vi "For Debug.vi"() -> ()   [LabVIEW 2015]
uses:
  AOP/Interface/CRDS/Controls/Ringdown Xctl/Ringdown.xctl
  Devices/Alicat/Session Based/Data/Alicat Data.lvclass
  Reusable/Data/Array Data/Single 1-D/Single_Array.lvclass
  Devices/TE Cooler/Data/TECData.lvclass
  Devices/TE Cooler/Data/TECData.lvclass/TECData.ctl
  Reusable/CRDS/Data/Main/CRDS Data.lvclass
  Reusable/CRDS/Data/Cell/CRDS Cell Data.lvclass/CRDS Cell Data.ctl
  Reusable/PAS/Data/Main/PAS Data.lvclass
  Reusable/PAS/Data/Cell/PAS Cell Data.lvclass
  Devices/TE Cooler/Data/Data Access/Read Input 1.vi
  Devices/TE Cooler/Data/Data Access/Read Input 2.vi
  Devices/TE Cooler/Data/Data Access/Read Power.vi
  Reusable/CRDS/Data/Cell/Read extParam.vi
  Reusable/CRDS/Data/Main/Read filter.vi
  Reusable/CRDS/Data/Main/Read CellData.vi
  Reusable/Data/Read measTime.vi
  Reusable/CRDS/Data/Cell/Read Ringdowns.vi
  Reusable/PAS/Data/Main/Write Current Cell.vi
  Reusable/PAS/Data/Main/Read Cell Frequency Data.vi
  Reusable/PAS/Data/Main/Read Cell Laser Diode Signal.vi
  Reusable/PAS/Data/Main/Read Cell Microphone Signal.vi
  Reusable/PAS/Data/Main/Read O3 flag.vi
  Reusable/PAS/Data/Main/Read CellData.vi
  Reusable/PAS/Data/Cell/Read derived.vi
  Reusable/Data/Array Data/Single 1-D/Read Data.vi
  Reusable/CRDS/Data/Cell/CRDS Cell Data.lvclass
panel:
  in  "Tab Control":enum32{"CRDS", "PAS", "TEC", "Housekeeping"}(tab)
  in  "PMT":bool
  in  "Rep Rate":i32(ring)=250 items=["1000"=1000, "500"=500, "250"=250]
  out "max":cluster{"[0]":sgl, "[1]":sgl}(graph)
  out "tau":cluster{"[0]":dbl, "[1]":dbl}(graph)
  out "Cell 1":T1 {"max" format="%#.6g"; "Tau0" format="%#.6g"; "TauCorr" format="%#.6g"; "etau" format="%#.6g"; "stdDevtau" format="%#.6g"; "extCorr" format="%#.6g"; "ext" format="%#.6g"; "Tau0Corr" format="%#.6g"; "Tau" format="%#.6g"}
  out "Cell 0":T1 {"max" format="%#.6g"; "Tau0" format="%#.6g"; "TauCorr" format="%#.6g"; "etau" format="%#.6g"; "stdDevtau" format="%#.6g"; "extCorr" format="%#.6g"; "ext" format="%#.6g"; "Tau0Corr" format="%#.6g"; "Tau" format="%#.6g"}
  in  "Num Samples per Cycle":dbl
  out "Ringdown":i16[][][](xcontrol)
  out "CRDS Time":timestamp format="%<%H:%M:%S%2u>T"
  out "Phase":dbl(graph)
  out "PAS Time":timestamp format="%<%H:%M:%S%2u>T"
  out "f0":sgl(graph)
  out "IA":sgl(graph)
  out "PAS Data":T2
  in  "Chirp Bandwidth":i16
  in  "Chirp fcenter":i16
  out "Laser Diode":waveform(i16)(graph)
  out "Frequency":waveform(sgl)(graph)
  out "Microphone":waveform(i16)(graph)
  in  "f0":dbl
  in  "DC":dbl
  in  "Vrange":dbl
  in  "Voffset":dbl
  in  "VspkParam":dbl[](array[numeric])
  in  "Speaker":bool
  in  "Modulation":dbl
  out "O3 Flag":bool
  in  "PAS TEC Power":bool
  in  "Main TEC Power":bool
  out "TEC Out":cluster{"[0]":sgl, "[1]":sgl}(graph)
  out "PAS":T3
  out "Main":T3
  in  "Tpas":sgl
  in  "Tmain":sgl
  in  "FanIn":bool
  in  "Alicat Names":string[](array[string])=["Pressure", "PAS", "CRD1", "Purge", "Ozone"]
  out "RH":cluster{"Numeric":sgl, "Numeric":sgl}(graph)
  out "T":cluster{"Numeric":sgl, "Numeric":sgl}(graph)
  out "P":T4(graph)
  in  "Solenoid  In":u8
  out "PPT 3":cluster{"P":dbl, "T":dbl}
  out "PPT 2":cluster{"P":dbl, "T":dbl}
  out "PPT 1":cluster{"P":dbl, "T":dbl}
  out "PAS":cluster{"RH":dbl, "T":dbl, "Td":dbl}
  out "CRD":cluster{"RH":dbl, "T":dbl, "Td":dbl}
  in  "Qsp":dbl[](array[numeric])
  in  "Pump":bool
  in  "Filter":bool
  out "Filter Out":bool
  out "Alicat Data":sgl[][](array[numeric])
  # "Number of samples in a single cylce refers to the number of samples that will be acquired during a ringdown.  The data acquisition is at 1 MHz, so if the value is 500, then the system is acquiring 500 us of samples per ringdown."
  # "The Rep Rate actually refers to the number of clock ticks between ringdowns.  The clock rate is 1 MHz, so if the value is 1000, there is 1000 us between each ringdown and laser is modulating at 1 kHz.  If the value is 2000,  then there are 2000 us between ringdowns and the laser is modulating at 500 Hz."
  # "Laser"
  # "Speaker"
  # "Alicat's are currently entered as follows:\nID                 Address   Controller?   Type                 Range\nPressure          A                Y                  Pressure           0-1000 \nPAS                  D                Y                  Mass                 0-5\nCRD1                B                Y                  Mass                 0-1\nPurge               E                Y                   Mass                 0-100\nOzone              F                 Y                  Volumetric       0-5"
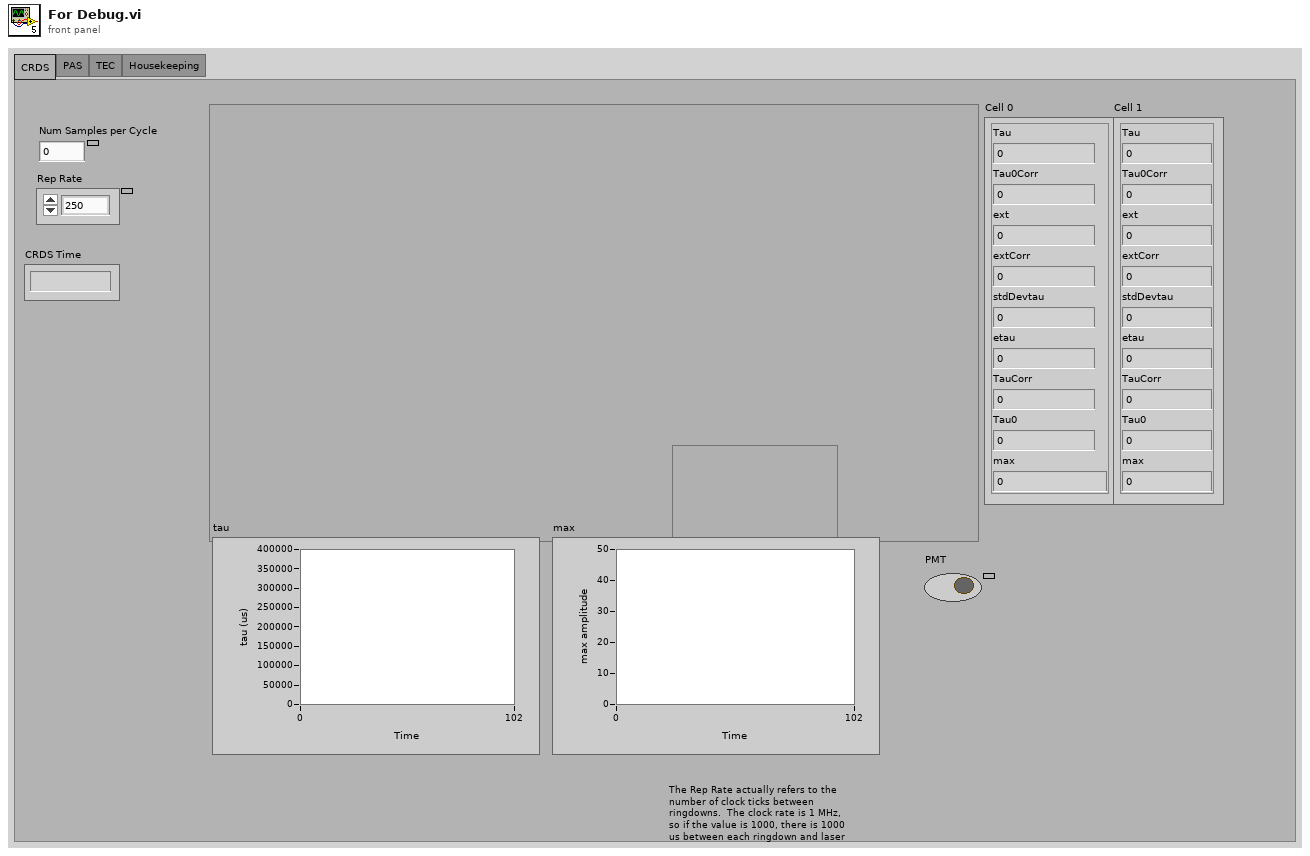
[diagram p1: front panel]
types:
  T1 = cluster{"Tau":dbl, "Tau0Corr":dbl, "ext":dbl, "extCorr":dbl, "stdDevtau":dbl, "etau":dbl, "TauCorr":dbl, "Tau0":dbl, "max":dbl}
  T2 = cluster{"f0 (Hz":dbl, "IA":dbl, "Noise Limit":dbl, "Q":dbl, "phase":dbl}
  T3 = cluster{"Input 1":dbl, "Input 2":dbl, "Power":dbl}
  T4 = cluster{"Numeric":sgl, "Numeric":sgl, "Numeric":sgl}
  T5 = cluster{"f0":sgl, "IA":sgl, "Q":sgl, "max":dbl[], "deltaPhi":dbl, "tau":dbl, "noiseLim":dbl, "ext":dbl}
  T6 = cluster{"f0":sgl, "IA":sgl, "noiseLim":dbl, "Q":sgl, "deltaPhi":dbl}
  T7 = typedef "extparam.ctl" = cluster{"Tau":sgl, "Tau0cor":sgl, "ext":sgl, "extCorr":sgl, "stdevTau":sgl, "eTau":sgl, "taucorr":sgl, "Tau0":sgl, "max":sgl}
  T8 = cluster{"Data Access:Input 1":sgl, "Data Access:Input 2":sgl, "Data Access:Power":sgl}
  T9 = cluster{"Data[0]":sgl, "Data[1]":sgl, "Data[2]":sgl}
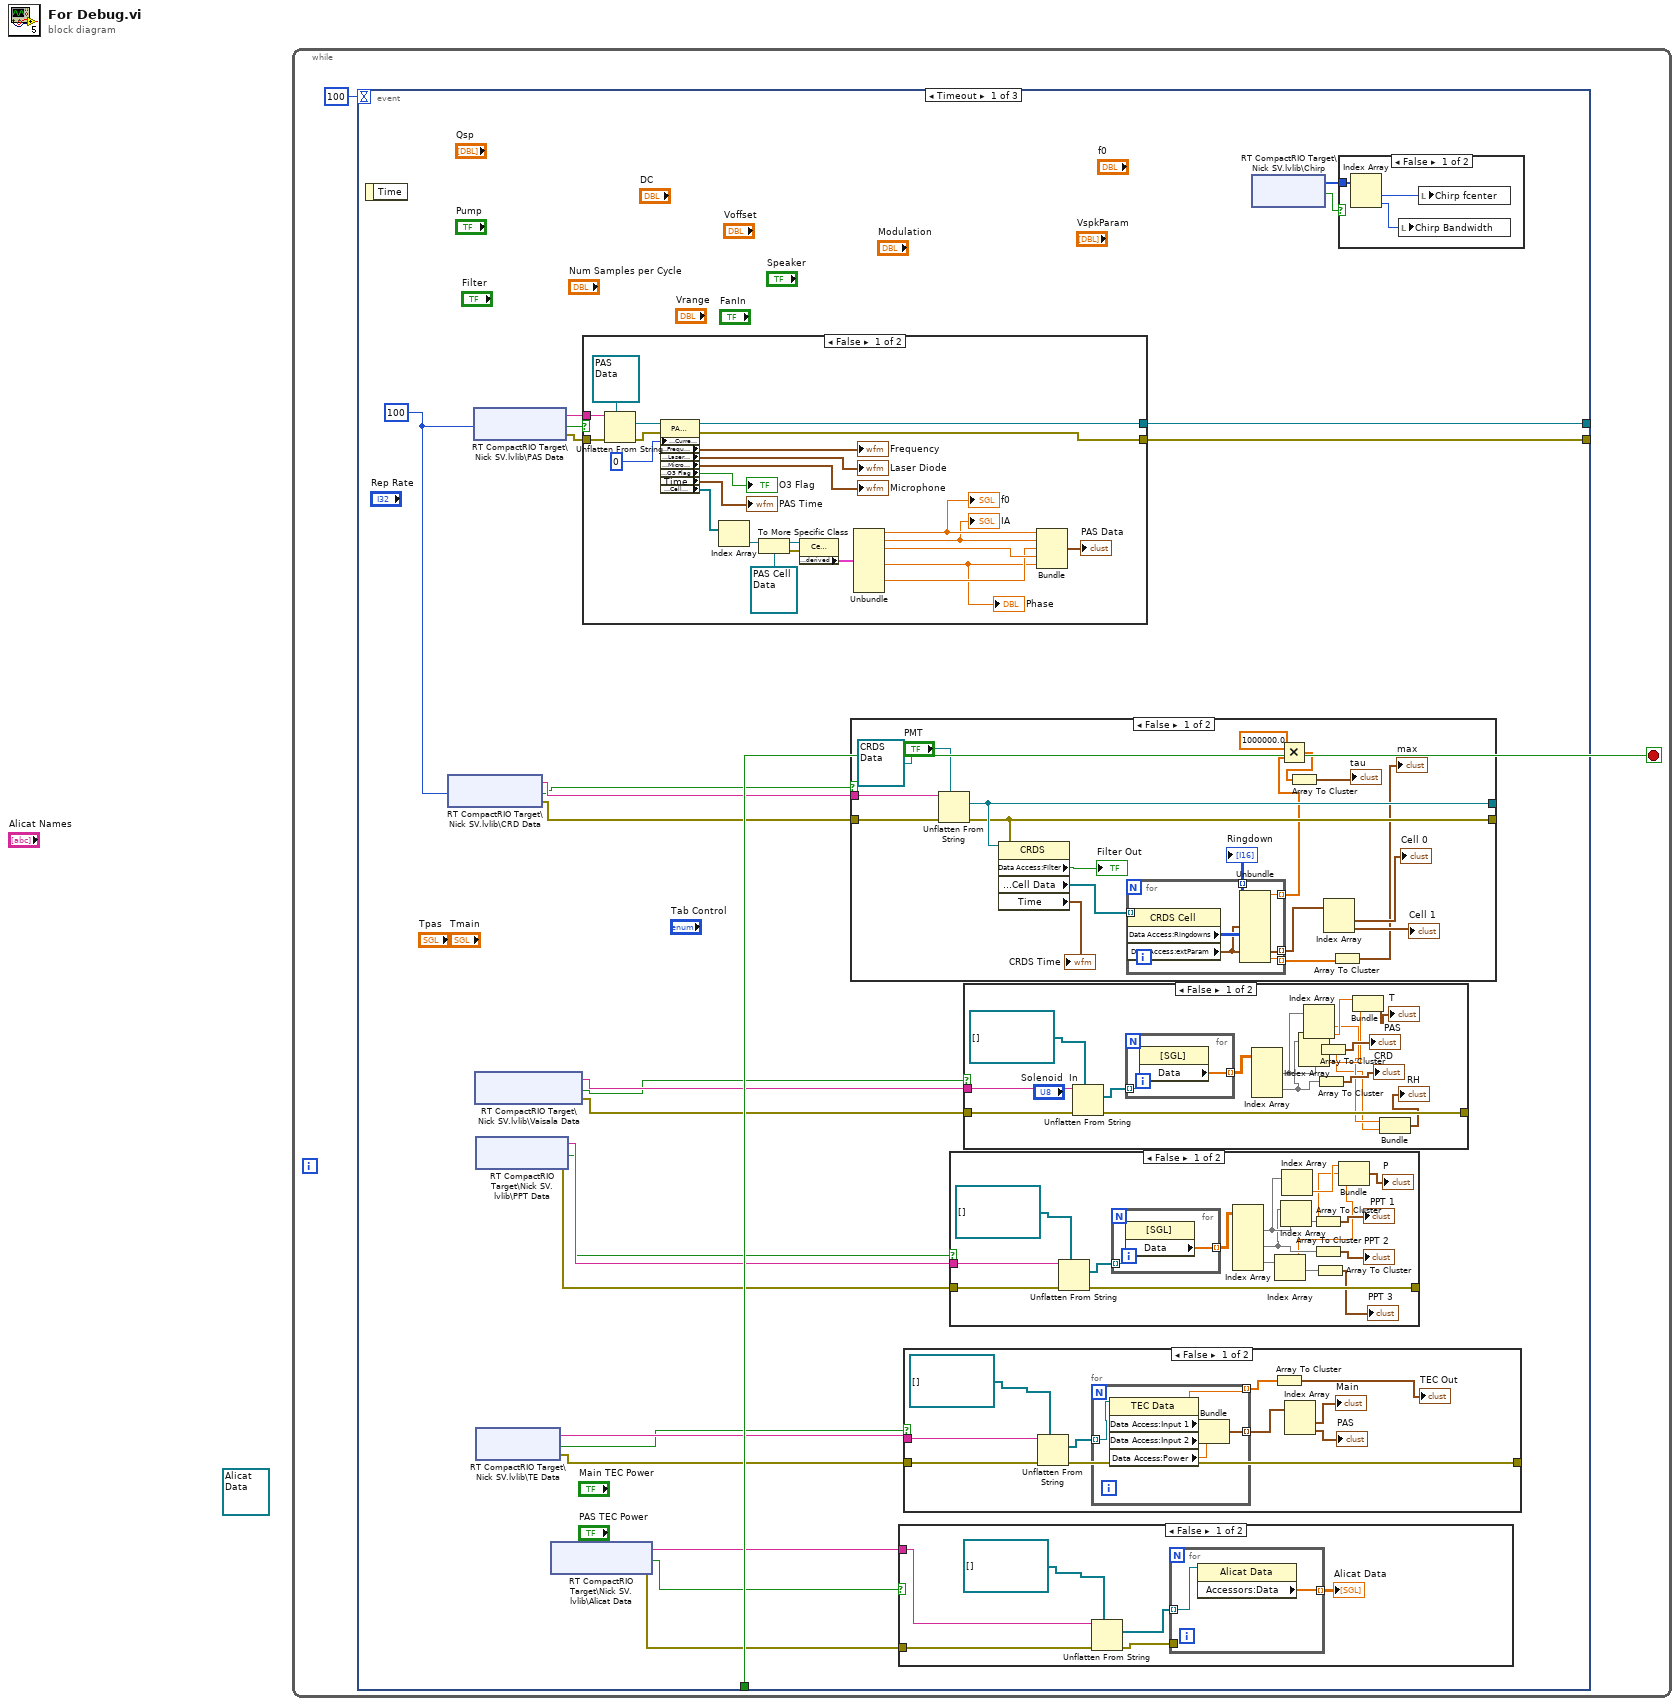
[diagram p0: block diagram]
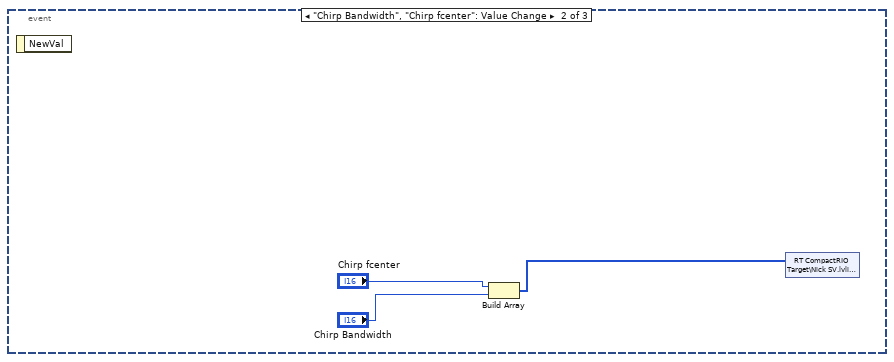
[diagram p9: hidden frame]
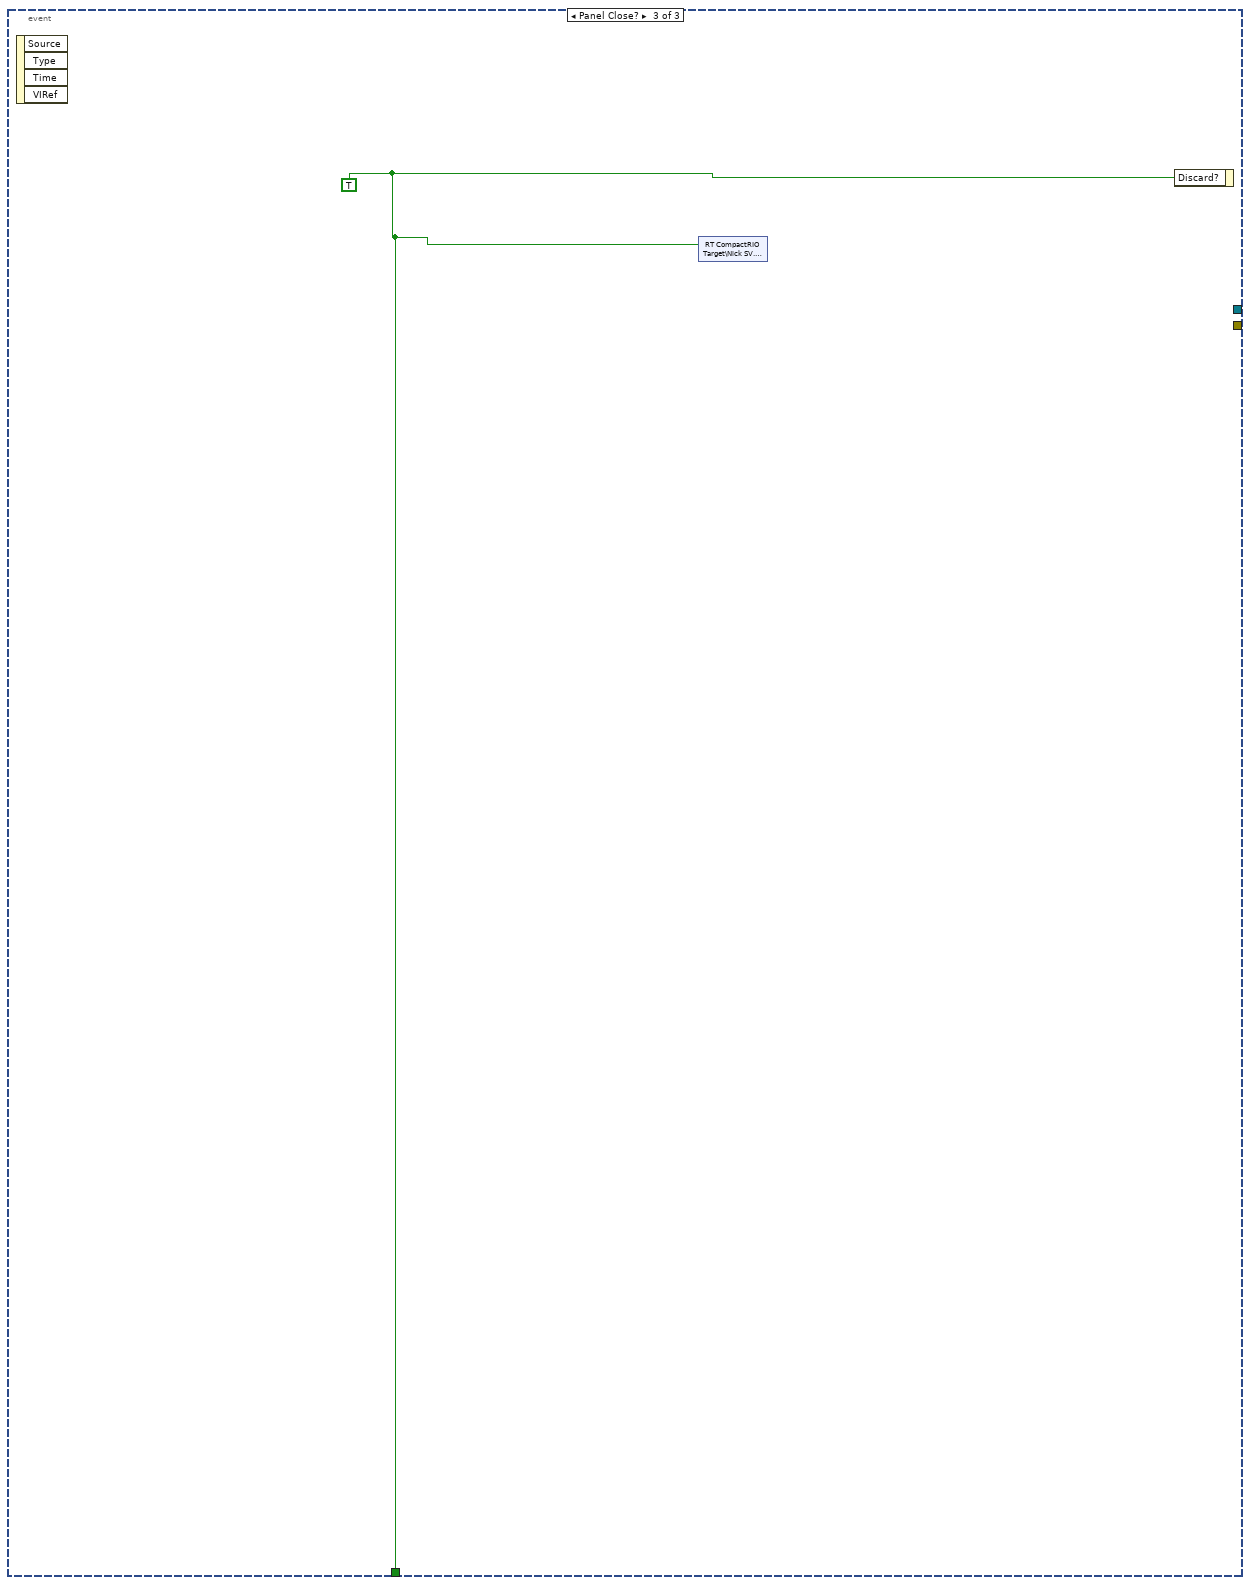
[diagram p10: hidden frame]
diagram:
  (unwired) refnum<class "Alicat Data.lvclass"> refnum ("Alicat Data")
  n1 = while {
    stop <- w2 stop-if-true
    n2 = event shown="[0] Timeout" {
      selector: _ -> [_ _ _]
      dyn-events: _ -> [_ _ _]
      timeout: 100 -> [_ _ _]
      tunnel: [_ _ w144] -> w2
      tunnel: [w24 _ _] -> _
      tunnel: [w23 _ _] -> _
      event Timeout {
        w17 = 100 ("ms timeout (0)")
        n3 = event-data() -> ()  [unwired: 1 in, 1 out]
        n4 = shared-variable "RT CompactRIO Target\\Nick SV.lvlib\\CRD Data"(w17) -> (w20:string, error out=w18:errorcluster, w19:bool)  [unwired: 1 in]
        n5 = shared-variable "RT CompactRIO Target\\Nick SV.lvlib\\PAS Data"(w17) -> (w25:string, error out=w22:errorcluster, w21:bool)  [unwired: 1 in]
        n6 = shared-variable "RT CompactRIO Target\\Nick SV.lvlib\\Vaisala Data"() -> (w16:string, error out=w14:errorcluster, w15:bool)  [unwired: 2 in]
        n7 = shared-variable "RT CompactRIO Target\\Nick SV.lvlib\\PPT Data"() -> (w13:string, error out=w11:errorcluster, w12:bool)  [unwired: 2 in]
        n8 = shared-variable "RT CompactRIO Target\\Nick SV.lvlib\\TE Data"() -> (w10:string, error out=w9:errorcluster, w8:bool)  [unwired: 2 in]
        n9 = shared-variable "RT CompactRIO Target\\Nick SV.lvlib\\Alicat Data"() -> (w5:string, error out=w3:errorcluster, w4:bool)  [unwired: 2 in]
        n10 = case shown="False" w21 {
          tunnel: w25 -> [w139 _]
          tunnel: [w133 _] -> w24
          tunnel: [w132 w140] -> w23
          tunnel: w22 -> [w138 w140]
          frame False {
            n11 = Unflatten From String(type=refnum<class "PAS Data.lvclass"> refnum ("PAS Data"), binary string=w139, error in (no error)=w138) -> (value=w136:refnum<class "PAS Data.lvclass">, error out=w135:errorcluster)  [unwired: 2 in, 1 out]
            n12 = property class="PAS Data"(reference=w136, error in=w135, "Data Access:Current Cell"=0 ("Current Cell")) -> (reference out=w133:refnum<class "PAS Data.lvclass">, error out=w132:errorcluster, "Data Access:Frequency"=→"Frequency":waveform(sgl), "Data Access:Laser Diode"=→"Laser Diode":waveform(i16), "Data Access:Microphone"=→"Microphone":waveform(i16), "Data Access:O3 Flag"=→"O3 Flag":bool, "Time"=→"PAS Time":timestamp, "Data Access:Cell Data"=w126:refnum<class "PAS Cell Data.lvclass">[])
            n13 = Index Array(array=w126) -> (element=w125:refnum<class "PAS Cell Data.lvclass">)  [unwired: 1 in]
            n14 = To More Specific Class(target class=refnum<class "PAS Cell Data.lvclass"> refnum ("Cell Data"), reference=w125) -> (specific class reference=w122:refnum<class "PAS Cell Data.lvclass">, error out=w123:errorcluster)  [unwired: 1 in]
            n15 = property class="Cell Data"(reference=w122, error in=w123) -> ("Data Access:derived"=w121:T5)  [unwired: 2 out]
            n16 = Unbundle(w121) -> ("f0"=w118:sgl, "IA"=w117:sgl, "Q"=w119:sgl, "deltaPhi"=w115:dbl, "noiseLim"=w116:dbl)  [unwired: 3 out]
            "f0" <- w118
            "IA" <- w117
            "Phase" <- w115
            n17 = Bundle("f0"=w118, "IA"=w117, "noiseLim"=w116, "Q"=w119, "deltaPhi"=w115) -> (→"PAS Data":T6)  [unwired: 1 in]
          }
          frame True {
          }
        }
        n18 = case shown="False" w19 {
          tunnel: w20 -> [w108 _]
          tunnel: [w105 _] -> _
          tunnel: [w104 w114] -> _
          tunnel: w18 -> [w107 w114]
          frame False {
            n19 = Unflatten From String(type=refnum<class "CRDS Data.lvclass"> refnum ("CRDS"), binary string=w108, error in (no error)=w107) -> (value=w105:refnum<class "CRDS Data.lvclass">, error out=w104:errorcluster)  [unwired: 2 in, 1 out]
            n20 = property class="CRDS"(reference=w105, error in=w104) -> ("Data Access:Filter"=→"Filter Out":bool, "Data Access:Cell Data"=w102:refnum<class "CRDS Cell Data.lvclass">[], "Time"=→"CRDS Time":timestamp)  [unwired: 2 out]
            n21 = for {
              tunnel: w102 -> [w113] mode=indexing
              tunnel: [w112] -> w101 mode=indexing
              tunnel: [w111] -> w99 mode=indexing
              tunnel: [w110] -> w93 mode=indexing
              tunnel: [w109] -> w95 mode=indexing
              n22 = property class="CRDS Cell"(reference=w113) -> ("Data Access:Ringdowns"=w112:i16[][], "Data Access:extParam"=w111:T7)  [unwired: 1 in, 2 out]
              n23 = Unbundle(w111) -> ("Tau"=w110:sgl, "max"=w109:sgl)  [unwired: 7 out]
            }
            "Ringdown" <- w101
            n24 = Multiply(x=1000000.0, y=w93) -> (x*y=w91:dbl[])
            n25 = Array To Cluster(array=w91) -> (cluster=→"tau":cluster{"[0]":dbl, "[1]":dbl})
            n26 = Index Array(array=w99) -> (element #1=→"Cell 0":T7, element #2=→"Cell 1":T7)  [unwired: 2 in]
            n27 = Array To Cluster(array=w95) -> (cluster=→"max":cluster{"[0]":sgl, "[1]":sgl})
          }
          frame True {
          }
        }
        n28 = case shown="False" w4 {
          tunnel: w5 -> [w30 _]
          tunnel: w3 -> [w29 _]
          frame False {
            n29 = Unflatten From String(type=refnum<class "Alicat Data.lvclass">[] [] ("TE Data"), binary string=w30, error in (no error)=w29) -> (value=w28:refnum<class "Alicat Data.lvclass">[], error out=w26:errorcluster)  [unwired: 2 in, 1 out]
            n30 = for {
              tunnel: w28 -> [w33] mode=indexing
              tunnel: [w32] -> w27 mode=indexing
              tunnel: w26 -> [_]
              n31 = property class="Alicat Data"(reference=w33) -> ("Accessors:Data"=w32:sgl[])  [unwired: 1 in, 2 out]
            }
            "Alicat Data" <- w27
          }
          frame True {
          }
        }
        n32 = case shown="False" w8 {
          tunnel: w10 -> [w46 _]
          tunnel: [w45 w52] -> _
          tunnel: w9 -> [w44 w52]
          frame False {
            n33 = Unflatten From String(type=refnum<class "TECData.lvclass">[] [] ("TE Data"), binary string=w46, error in (no error)=w44) -> (value=w43:refnum<class "TECData.lvclass">[], error out=w45:errorcluster)  [unwired: 2 in, 1 out]
            n34 = for {
              tunnel: w43 -> [w51] mode=indexing
              tunnel: [w48] -> w41 mode=indexing
              tunnel: [w47] -> w38 mode=indexing
              n35 = property class="TEC Data"(reference=w51) -> ("Data Access:Input 1"=w47:sgl, "Data Access:Input 2"=w50:sgl, "Data Access:Power"=w49:sgl)  [unwired: 1 in, 2 out]
              n36 = Bundle("Data Access:Input 1"=w47, "Data Access:Input 2"=w50, "Data Access:Power"=w49) -> (w48:T8)  [unwired: 1 in]
            }
            n37 = Array To Cluster(array=w38) -> (cluster=→"TEC Out":cluster{"[0]":sgl, "[1]":sgl})
            n38 = Index Array(array=w41) -> (element #1=→"Main":T8, element #2=→"PAS":T8)  [unwired: 2 in]
          }
          frame True {
          }
        }
        n39 = case shown="False" w12 {
          tunnel: w13 -> [w68 _]
          tunnel: [w67 w71] -> _
          tunnel: w11 -> [w66 w71]
          frame False {
            n40 = Unflatten From String(type=refnum<class "Single_Array.lvclass">[] [], binary string=w68, error in (no error)=w66) -> (value=w64:refnum<class "Single_Array.lvclass">[], error out=w67:errorcluster)  [unwired: 2 in, 1 out]
            n41 = for {
              tunnel: w64 -> [w70] mode=indexing
              tunnel: [w69] -> w63 mode=indexing
              n42 = property class="[SGL]"(reference=w70) -> ("Data"=w69:sgl[])  [unwired: 1 in, 2 out]
            }
            n43 = Index Array(array=w63) -> (element #1=w59:sgl[], element #2=w58:sgl[], element #3=w57:sgl[])  [unwired: 6 in]
            n44 = Index Array(array=w57) -> (element=w54:sgl)  [unwired: 1 in]
            n45 = Index Array(array=w58) -> (element=w55:sgl)  [unwired: 1 in]
            n46 = Index Array(array=w59) -> (element=w56:sgl)  [unwired: 1 in]
            n47 = Array To Cluster(array=w59) -> (cluster=→"PPT 1":cluster{"Data[0]":sgl, "Data[1]":sgl})
            n48 = Array To Cluster(array=w58) -> (cluster=→"PPT 2":cluster{"Data[0]":sgl, "Data[1]":sgl})
            n49 = Array To Cluster(array=w57) -> (cluster=→"PPT 3":cluster{"Data[0]":sgl, "Data[1]":sgl})
            n50 = Bundle("Numeric"=w56, "Numeric"=w55, "Numeric"=w54) -> (→"P":T4)  [unwired: 1 in]
          }
          frame True {
          }
        }
        n51 = case shown="False" w15 {
          tunnel: w16 -> [w87 _]
          tunnel: [w86 w90] -> _
          tunnel: w14 -> [w85 w90]
          frame False {
            n52 = Unflatten From String(type=refnum<class "Single_Array.lvclass">[] [], binary string=w87, error in (no error)=w85) -> (value=w83:refnum<class "Single_Array.lvclass">[], error out=w86:errorcluster)  [unwired: 2 in, 1 out]
            n53 = for {
              tunnel: w83 -> [w89] mode=indexing
              tunnel: [w88] -> w82 mode=indexing
              n54 = property class="[SGL]"(reference=w89) -> ("Data"=w88:sgl[])  [unwired: 1 in, 2 out]
            }
            n55 = Index Array(array=w82) -> (element #1=w79:sgl[], element #2=w78:sgl[])  [unwired: 4 in]
            n56 = Index Array(array=w78) -> (element #1=w73:sgl, element #2=w76:sgl)  [unwired: 2 in]
            n57 = Index Array(array=w79) -> (element #1=w74:sgl, element #2=w77:sgl)  [unwired: 2 in]
            n58 = Array To Cluster(array=w78) -> (cluster=→"CRD":T9)
            n59 = Array To Cluster(array=w79) -> (cluster=→"PAS":T9)
            n60 = Bundle("Numeric"=w77, "Numeric"=w76) -> (→"T":cluster{"Numeric":sgl, "Numeric":sgl})  [unwired: 1 in]
            n61 = Bundle("Numeric"=w74, "Numeric"=w73) -> (→"RH":cluster{"Numeric":sgl, "Numeric":sgl})  [unwired: 1 in]
          }
          frame True {
          }
        }
        n62 = shared-variable "RT CompactRIO Target\\Nick SV.lvlib\\Chirp"() -> (w6:i16[], w7:bool)  [unwired: 2 in, 1 out]
        n63 = case shown="False" w7 {
          tunnel: w6 -> [w36 _]
          frame False {
            n64 = Index Array(array=w36) -> (element #1=w35:i16, element #2=w34:i16)  [unwired: 2 in]
            n65 = local write "Chirp Bandwidth"(w34) -> ()
            n66 = local write "Chirp fcenter"(w35) -> ()
          }
          frame True {
          }
        }
      }
      event "Chirp Bandwidth", "Chirp fcenter": Value Change {
        n67 = event-data() -> ()  [unwired: 1 in, 1 out]
        n68 = Build Array("Chirp fcenter", "Chirp Bandwidth") -> (w141:i16[])
        n69 = shared-variable "RT CompactRIO Target\\Nick SV.lvlib\\Chirp"(w141) -> ()  [unwired: 1 in, 1 out]
      }
      event Panel Close? {
        w144 = TRUE ("Discard?")
        n70 = event-data() -> ()  [unwired: 1 in, 4 out]
        n71 = shared-variable "RT CompactRIO Target\\Nick SV.lvlib\\Stop"(w144) -> ()  [unwired: 1 in, 1 out]
        n72 = event-data("Discard?"=w144) -> ()  [unwired: 1 in, 1 out]
      }
    }
  }
